vi "in.vi"(5 "IN VARIANT":variant, 7 "Ip":string, 9 "Name in":string, 11 "error in (no error)":errorcluster, 12 "timout":i32=-1) -> (6 "OUT VARIANT":variant, 10 "Valid data":bool, 15 "error out":errorcluster)   [LabVIEW 2015]
doc: "BLOCKING read of tuple \"name\" from tuple space"
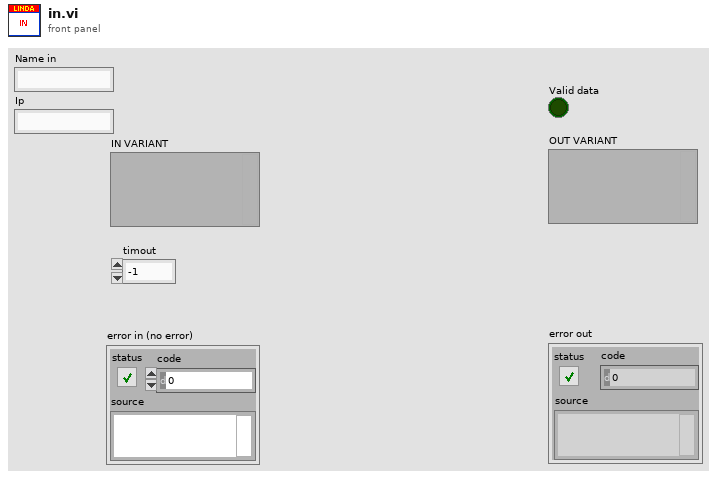
[diagram p1: front panel]
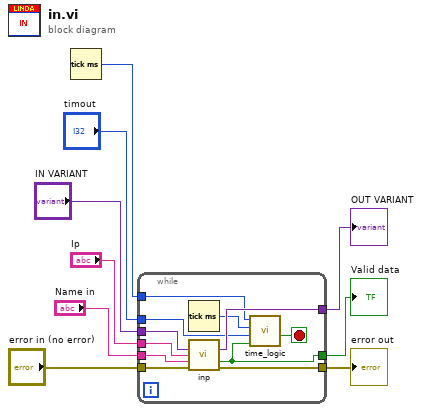
[diagram p0: block diagram]
diagram:
  n1 = Tick Count (ms)() -> (millisecond timer value=w5:u32)
  n2 = while {
    tunnel: "IN VARIANT" -> [w20]
    tunnel: [w19] -> w8
    tunnel: "error in (no error)" -> [w18]
    tunnel: [w17] -> w6
    tunnel: w5 -> [w16]
    tunnel: "timout" -> [w14]
    tunnel: [w12] -> w3
    tunnel: "Name in" -> [w11]
    tunnel: "Ip" -> [w10]
    stop <- w13 stop-if-true
    n3 = Tick Count (ms)() -> (millisecond timer value=w15:u32)
    n4 = call "inp.vi"("IN VARIANT"=w20, "Ip"=w10, "Name in"=w11, "error in (no error)"=w18) -> ("OUT VARIANT"=w19:variant, "Valid data"=w12:bool, "error out"=w17:errorcluster)  [unwired: 9 in]
    n5 = call "time_logic.vi"("Boolean in"=w12, "timout"=w14, "Elapsed Time"=w15, "Start Time"=w16) -> ("Boolean out"=w13:bool)  [unwired: 7 in]
  }
  "OUT VARIANT" <- w8
  "error out" <- w6
  "Valid data" <- w3
